vi "Save Devices.vi"(8 "error in":errorcluster) -> (0 "error out":errorcluster)   [LabVIEW 2024, in "Data Base.lvlib"]
uses:
  Data Base.lvlib
  Support/General Type Defs/Global Data.vi
  <vilib>/Utility/config.llb/Write Key (String).vi
  <vilib>/Utility/config.llb/NI_LVConfig.lvlib
  Support/General Type Defs/General Type Defs.lvlib
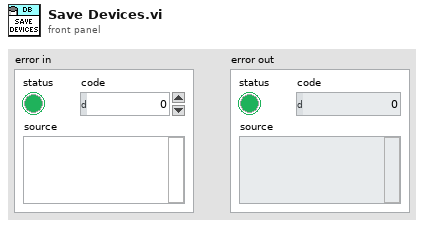
[diagram p1: front panel]
types:
  T1 = typedef "NI_LVConfig.lvlib/Config Data RefNum.ctl" = refnum<k1>
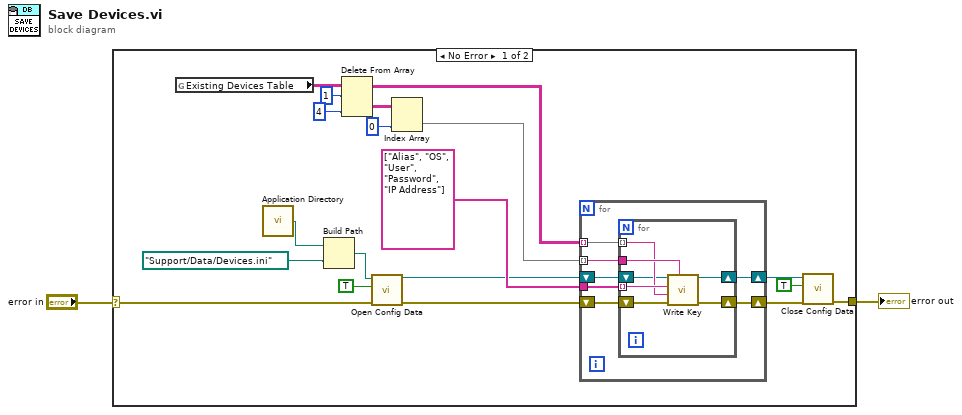
[diagram p0: block diagram]
diagram:
  n1 = case shown="No Error" "error in" {
    selector: "error in" -> [w3 w36]
    tunnel: [w7 w36] -> w2
    frame No Error {
      n2 = global read "Global Data.vi" "Existing Devices Table"() -> (w19:string[][])
      n3 = call <vilib>:"Application Directory.vi"() -> ("Application Directory"=w21:path)
      n4 = Build Path(base path=w21, name or relative path=path "Support/Data/Devices.ini") -> (appended path=w14:path)
      n5 = Delete From Array(array=w19, length=1, index (col)=4) -> (deleted portion=w16:string[][], array with subset deleted=w10:string[][])  [unwired: 1 in]
      n6 = call <vilib>:"Open Config Data.vi"("error in (no error)"=w3, "create file if necessary (T)"=TRUE, "configuration file path"=w14) -> ("error out"=w9:errorcluster, "refnum"=w5:T1)  [unwired: 6 in, 1 out]
      n7 = Index Array(array=w16, index (col)=0) -> (element=w12:string[])  [unwired: 1 in]
      n8 = for {
        tunnel: w12 -> [w28] mode=indexing
        tunnel: string[] ["Alias", "OS", "User", "Password", "IP Address"] -> [w27]
        tunnel: w10 -> [w26] mode=indexing
        shift-right: [w24] -> w8
        shift-left: w9 -> [w25]
        shift-right: [w23] -> w6
        shift-left: w5 -> [w22]
        n9 = for {
          tunnel: w28 -> [w35]
          tunnel: w27 -> [w34] mode=indexing
          tunnel: w26 -> [w33] mode=indexing
          shift-right: [w31] -> w24
          shift-left: w25 -> [w32]
          shift-right: [w30] -> w23
          shift-left: w22 -> [w29]
          n10 = call-poly <vilib>:"Write Key.vi"("section"=w35, "error in (no error)"=w32, "value"=w33, "key"=w34, "refnum"=w29) -> ("error out"=w31:errorcluster, "refnum out"=w30:T1)  [unwired: 4 in, 1 out]
        }
      }
      n11 = call <vilib>:"Close Config Data.vi"("error in (no error)"=w8, "write file if changed (T)"=TRUE, "refnum"=w6) -> ("error out"=w7:errorcluster)  [unwired: 7 in, 1 out]
    }
    frame Error {
    }
  }
  "error out" <- w2
